vi "Type Panel.vi"(11 "TextPanel in":refnum<class "TextPanel.lvclass">) -> ()   [LabVIEW 2020, in "Conditum-Tools.lvlib" / "TextPanel.lvclass"]
uses:
  TextPanel.lvclass
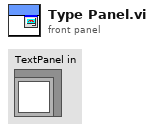
[diagram p1: front panel]
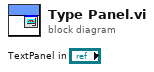
[diagram p0: block diagram]
diagram:
